vi "pmu_Extract Zero-crossing Frequencies.vi"(10 "timestamps in":dbl[](array[numeric]), 11 "frequencies in":dbl[](array[numeric])) -> (2 "zero-crossing timestamps":dbl[](array[numeric]), 3 "zero-crossing frequencies":dbl[](array[numeric]))   [LabVIEW 2013, in "NI_EP_PMU.lvlib"]
uses:
  <vilib>/addons/Electrical Power/PMU/NI_EP_PMU.lvlib
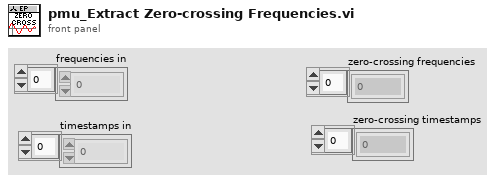
[diagram p1: front panel]
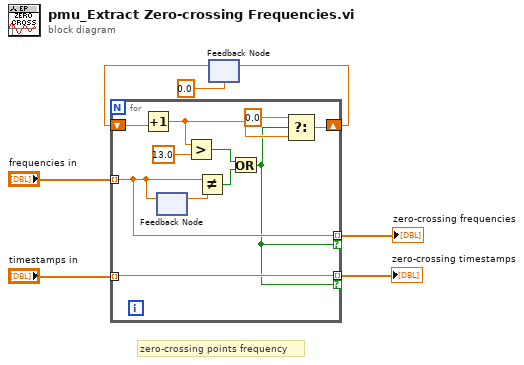
[diagram p0: block diagram]
diagram:
  # "zero-crossing points frequency"
  n1 = feedback #1(0.0) -> (w3:dbl)
  n2 = for {
    tunnel: "frequencies in" -> [w9] mode=indexing
    tunnel: "timestamps in" -> [w10] mode=indexing
    shift-right: [w15] -> w5
    shift-left: w3 -> [w12]
    tunnel: [w10] -> w2 mode=indexing if=w8
    tunnel: [w9] -> w1 mode=indexing if=w8
    n3 = Increment(x=w12) -> (x+1=w11:dbl)
    n4 = feedback-in #2(w9) -> ()
    n5 = feedback #2() -> (w18:dbl)  [unwired: 1 in]
    n6 = Greater?(x=w11, y=13.0) -> (0:w14:bool)
    n7 = Not Equal?(x=w9, y=w18) -> (x != y?=w13:bool)
    n8 = Or(x=w14, y=w13) -> (x .or. y?=w8:bool)
    n9 = Select(t=0.0, s=w8, f=w11) -> (s? t:f=w15:dbl)
  }
  "zero-crossing frequencies" <- w1
  "zero-crossing timestamps" <- w2
  n10 = feedback-in #1(w5) -> ()
